vi "Timestamp2Posix.vi"(5 "timestamp":timestamp) -> (2 "POSIX":dbl format="%.6f")   [LabVIEW 2020]
panel:
  # "converts a LabVIEW timestamp to POSIX seconds since 1970-01-01 00:00:00"
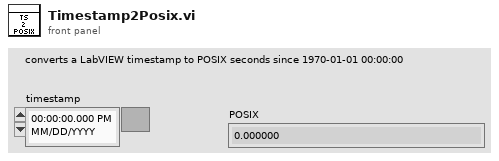
[diagram p1: front panel]
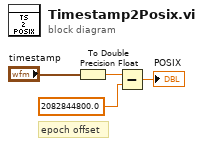
[diagram p0: block diagram]
diagram:
  # "epoch offset"
  n1 = To Double Precision Float(number="timestamp") -> (double precision float=w4:dbl)
  n2 = Subtract(x=w4, y=2082844800.0) -> (x-y=→"POSIX":dbl)
